vi "SW_Config.vi"(8 "error in (no error)":errorcluster, 10 "SW Config In":T1, 11 "Step":enum16{"Initial", "Write", "Read"}(ring)) -> (0 "error out":errorcluster, 2 "SW Config out":T1)   [LabVIEW 2017]
uses:
  Ctrls/TesterInfo.ctl
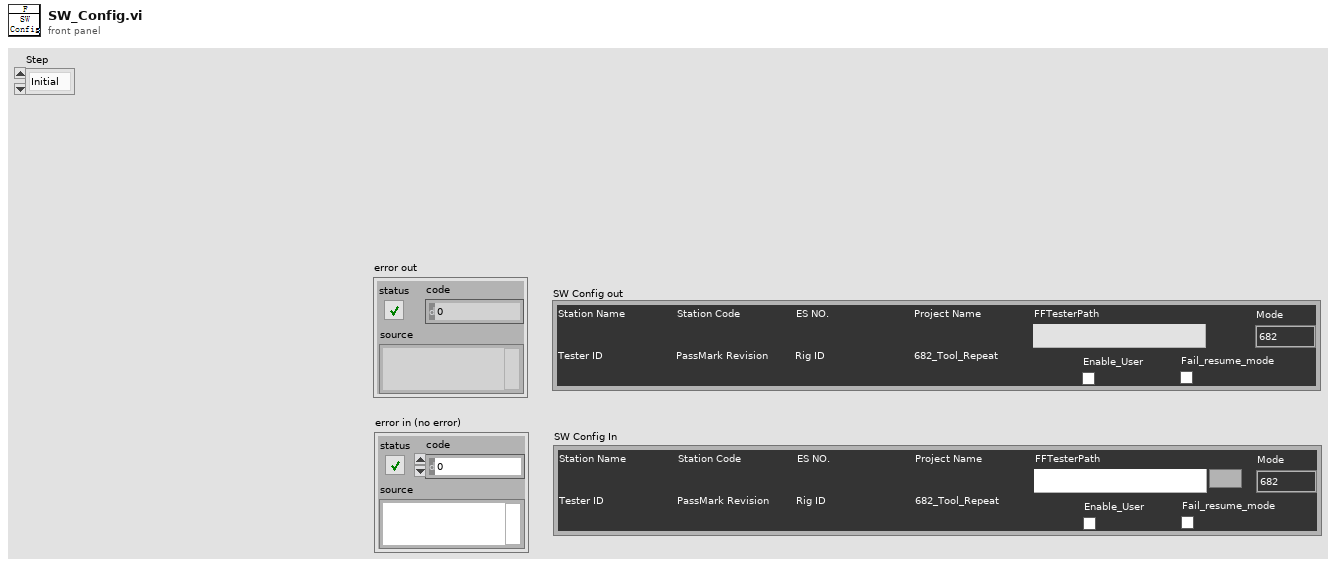
[diagram p1: front panel]
types:
  T1 = typedef "TesterInfo.ctl" = cluster{"Station Name":string, "Station Code":string, "ES NO.":string, "Tester ID":string, "PassMark Revision":string, "Rig ID":string, "682_Tool_Repeat":string, "Project Name":string, "FFTesterPath":path, "Enable_User":bool, "Mode":enum16{"682"}, "Fail_resume_mode":bool}
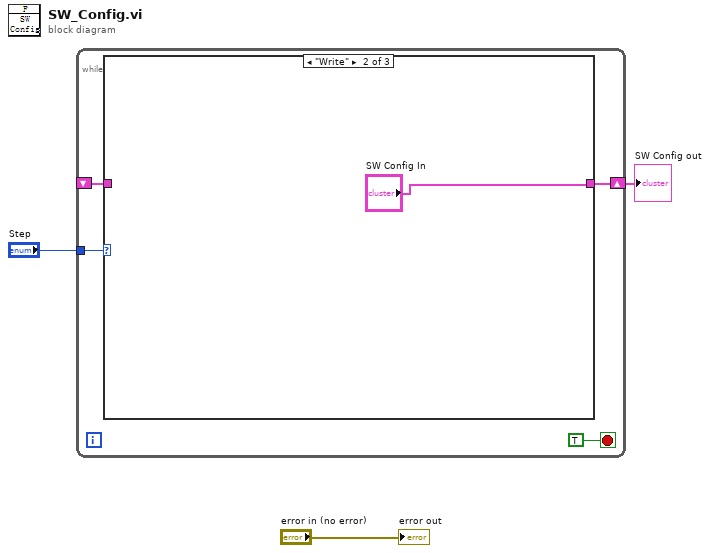
[diagram p0: block diagram]
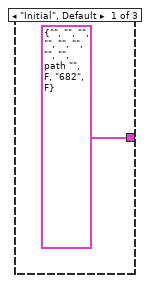
[diagram p2: hidden frame]
diagram:
  n1 = while {
    tunnel: "Step" -> [w6]
    shift-right: [w5] -> w1
    shift-left: _ -> [w4]
    stop <- TRUE stop-if-true
    n2 = case shown="\"Write\"" w6 {
      tunnel: [T1 {"Station Name"="", "Station Code"="", "ES NO."="", "Tester ID"="", "PassMark Revision"="", "Rig ID"="", "682_Tool_Repeat"="", "Project Name"="", "FFTesterPath"=path "", "Enable_User"=FALSE, "Mode"=enum."682", "Fail_resume_mode"=FALSE} ("SW Config In") "SW Config In" w10] -> w5
      tunnel: w4 -> [_ _ w10]
      frame "Initial", Default {
      }
      frame "Write" {
      }
      frame "Read" {
      }
    }
  }
  "SW Config out" <- w1
  "error out" <- "error in (no error)"
